vi "read TBM configuration.vi"(8 "error in":errorcluster, 11 "EthernetIP editor node in":refnum<class "EthernetIP editor node.lvclass">) -> (0 "error out":errorcluster, 2 "TBM configuration out":refnum<class "TBM configuration.lvclass">, 3 "EthernetIP editor node out":refnum<class "EthernetIP editor node.lvclass">)   [LabVIEW 2013, in "EthernetIP editor node.lvclass"]
uses:
  EthernetIP editor node.lvclass
  <vilib>/NI/Tag Bus Module Framework/root configuration/TBM configuration.lvclass
  EthernetIP editor node.lvclass/EthernetIP editor node.ctl
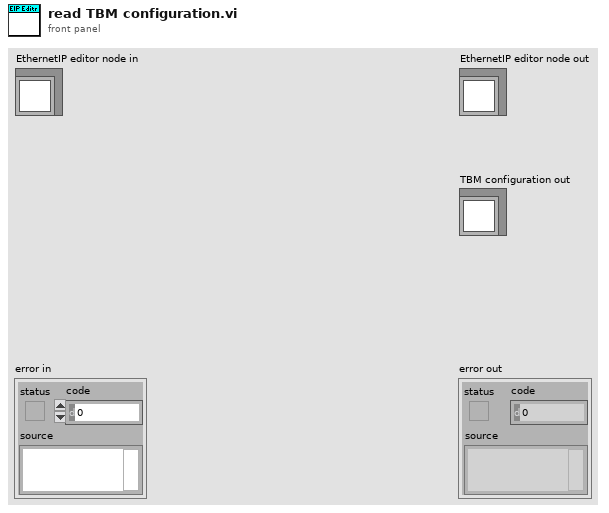
[diagram p1: front panel]
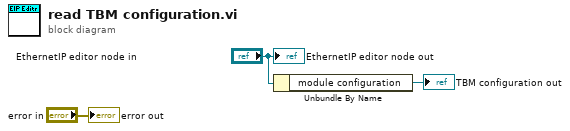
[diagram p0: block diagram]
diagram:
  n1 = Unbundle By Name("EthernetIP editor node in") -> ("module configuration"=→"TBM configuration out":refnum<class "EthernetIP configuration.lvclass">)
  "error out" <- "error in"
  "EthernetIP editor node out" <- "EthernetIP editor node in"
